vi "AdaptToInputs.vi"(3 "Term Types":T1, 4 "XRef":refnum<vi>, 5 "State In":T5) -> (0 "Reply":string[](array[string]), 2 "State Out":T5)   [LabVIEW 2018, in "Foreign Key Sort.xnode"]
uses:
  Foreign Key Sort.xnode
  State.ctl
  <vilib>/XNodeSupport/XNodeTermTypeIDPairs.ctl
  <vilib>/XNodeSupport/XNodeTermTypeIDPair.ctl
  <vilib>/XNodeSupport/XNodeType.ctl
  <vilib>/XNodeSupport/XNodeString.ctl
  <userlib>/_LAVAcr/Scripting Tools/XNode Support/TypeDefs/Array element Tests.ctl
  <userlib>/_LAVAcr/Scripting Tools/XNode Support/Find term type by ID_type.vi
  <userlib>/_LAVAcr/Scripting Tools/XNode Support/XNode Support.lvlib
  <vilib>/XNodeSupport/NI_XNodeSupport.lvlib
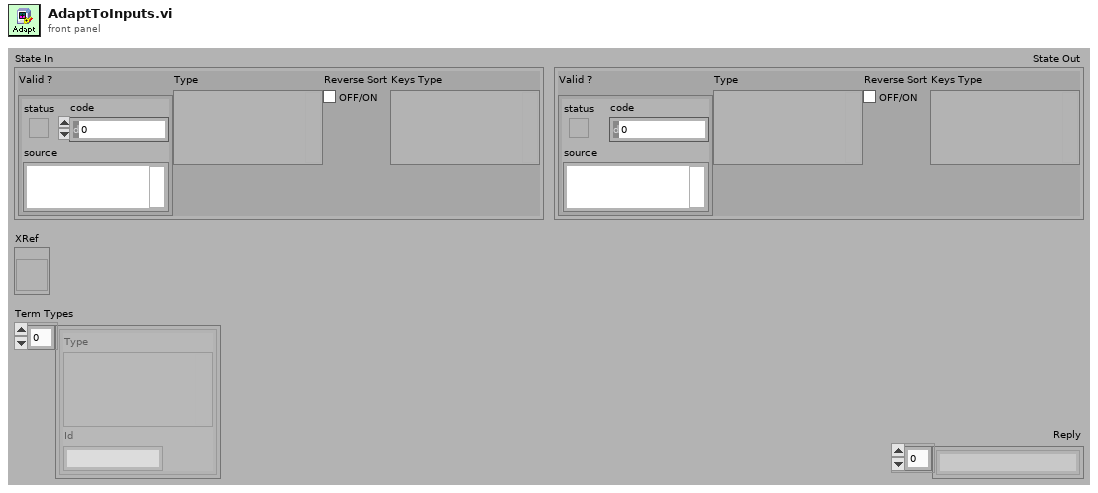
[diagram p1: front panel]
types:
  T1 = typedef "NI_XNodeSupport.lvlib/XNodeTermTypeIDPairs.ctl" = T2[]
  T2 = typedef "NI_XNodeSupport.lvlib/XNodeTermTypeIDPair.ctl" = cluster{"Type":T3, "Id":T4}
  T3 = typedef "NI_XNodeSupport.lvlib/XNodeType.ctl" = variant
  T4 = typedef "NI_XNodeSupport.lvlib/XNodeString.ctl" = string
  T5 = typedef "Foreign Key Sort.xnode/State.ctl" = cluster{"Valid ?":errorcluster, "Type":variant, "Reverse Sort":bool, "Keys Type":variant}
  T6 = enum16{"No Check", "At Least n dimensions", "Exactly N Dimensions"}
  T7 = typedef "Scripting Tools.lvlib/XNode Support.lvlib/Array element Tests.ctl" = enum16{"Any Element", "Numeric", "Integer", "Float", "Complex", "Boolean", "String", "Sortable"}
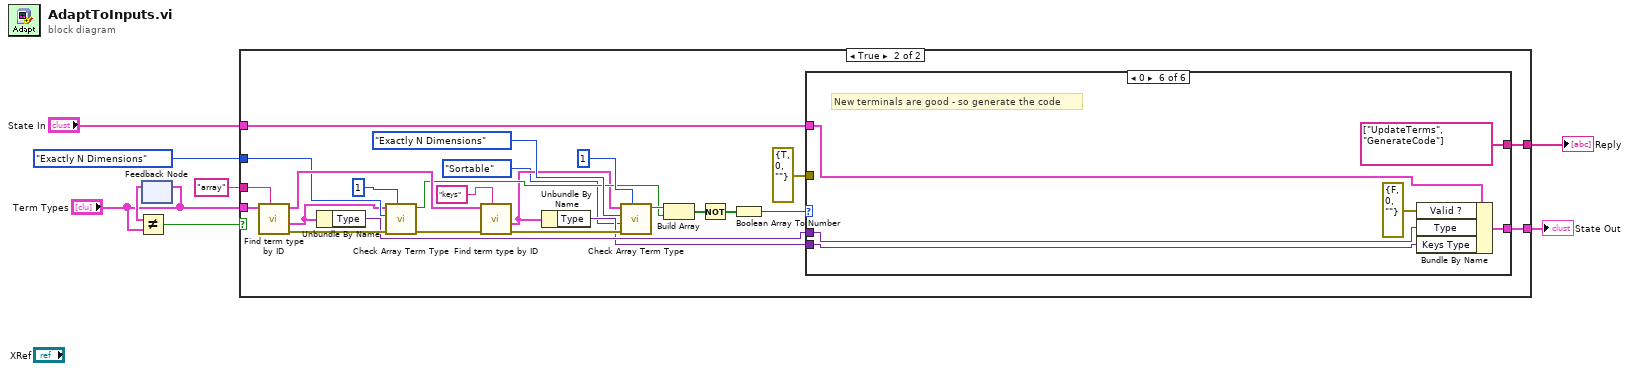
[diagram p0: block diagram]
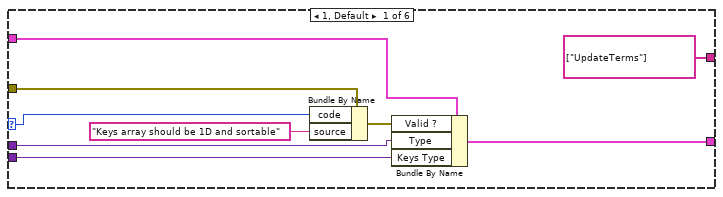
[diagram p3: hidden frame]
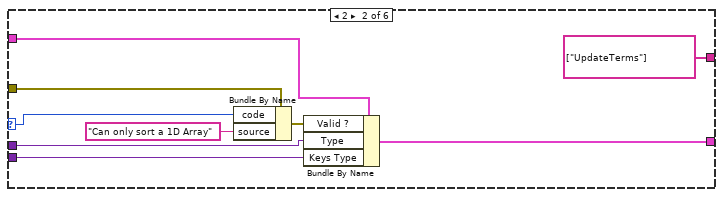
[diagram p4: hidden frame]
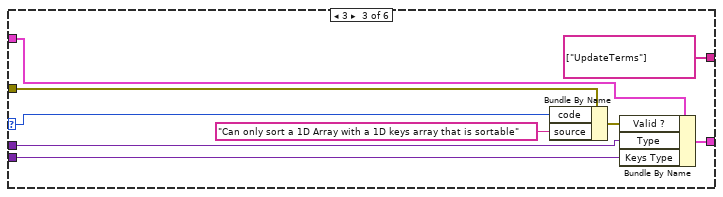
[diagram p5: hidden frame]
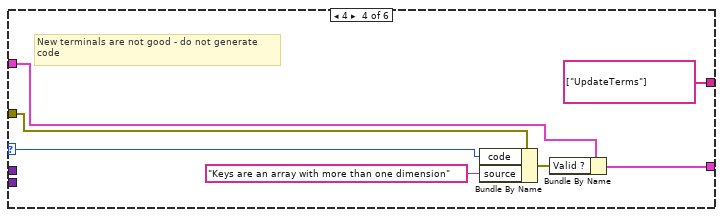
[diagram p6: hidden frame]
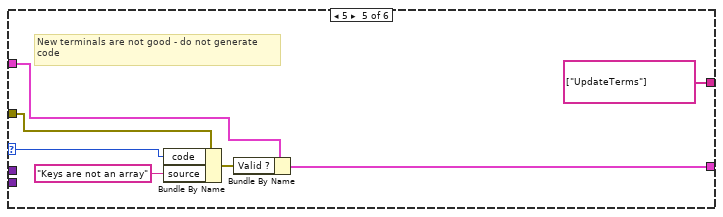
[diagram p7: hidden frame]
diagram:
  n1 = feedback-in #1("Term Types") -> ()
  n2 = feedback #1() -> (w4:T1)  [unwired: 1 out]
  n3 = Not Equal?(x=w4, y="Term Types") -> (x != y?=w1:bool)
  n4 = case shown="True" w1 {
    tunnel: [w9 w34] -> w8
    tunnel: [_ w33] -> w7
    tunnel: "array" ("Search ID") -> [_ w32]
    tunnel: T6."Exactly N Dimensions" ("Dimension Check") -> [_ w27]
    tunnel: "Term Types" -> [_ w11]
    tunnel: "State In" -> [w9 w10]
    frame False {
    }
    frame True {
      n5 = call-poly <userlib>:"Find term type by ID.vi"("Search ID"=w32, "Term Types"=w11) -> ("error out"=w28:errorcluster, "Term Type"=w16:T2, "Other Term Types"=w31:T2[])  [unwired: 1 in, 6 out]
      n6 = Unbundle By Name(w16) -> ("Type"=w15:T3)
      n7 = call <userlib>:"Check Array Term Type.vi"("Dimensions Required"=1, "error in (no error)"=w28, "Dimension Check"=w27, "Term Type"=w16) -> ("error out"=w25:errorcluster, "Is Good ?"=w20:bool)  [unwired: 1 in, 5 out]
      n8 = call-poly <userlib>:"Find term type by ID.vi"("Search ID"="keys", "error in (no error)"=w25, "Term Types"=w31) -> ("error out"=w24:errorcluster, "Term Type"=w14:T2)  [unwired: 7 out]
      n9 = Unbundle By Name(w14) -> ("Type"=w13:T3)
      n10 = call <userlib>:"Check Array Term Type.vi"("Dimensions Required"=1, "error in (no error)"=w24, "Element Check"=Array_element_Tests."Sortable", "Dimension Check"=T6."Exactly N Dimensions", "Term Type"=w14) -> ("Is Good ?"=w21:bool)  [unwired: 6 out]
      n11 = Build Array(w21, w20) -> (w19:bool[])
      n12 = Not(x=w19) -> (.not. x?=w18:bool[])
      n13 = Boolean Array To Number(Boolean array=w18) -> (number=w17:u32)
      n14 = case shown="0" w17 {
        selector: w17 -> [w37 w46 w55 w62 w69 _]
        tunnel: w10 -> [w43 w52 w61 w68 w75 w81]
        tunnel: [w42 w51 w60 w67 w74 w79] -> w34
        tunnel: [string[] ["UpdateTerms"] ("Reply") string[] ["UpdateTerms"] ("Reply") string[] ["UpdateTerms"] ("Reply") string[] ["UpdateTerms"] ("Reply") string[] ["UpdateTerms"] ("Reply") string[] ["UpdateTerms", "GenerateCode"] ("Reply")] -> w33
        tunnel: errorcluster {"status"=TRUE, "code"=0, "source"=""} ("Valid ?") -> [w40 w49 w58 w65 w72 _]
        tunnel: w13 -> [w35 w44 w53 _ _ w77]
        tunnel: w15 -> [w36 w45 w54 _ _ w76]
        frame 1, Default {
          n15 = Bundle By Name(cluster=w40, "code"=w37, "source"="Keys array should be 1D and sortable") -> (w39:errorcluster)
          n16 = Bundle By Name(cluster=w43, "Valid ?"=w39, "Type"=w36, "Keys Type"=w35) -> (w42:T5)
        }
        frame 2 {
          n17 = Bundle By Name(cluster=w49, "code"=w46, "source"="Can only sort a 1D Array") -> (w48:errorcluster)
          n18 = Bundle By Name(cluster=w52, "Valid ?"=w48, "Type"=w45, "Keys Type"=w44) -> (w51:T5)
        }
        frame 3 {
          n19 = Bundle By Name(cluster=w58, "code"=w55, "source"="Can only sort a 1D Array with a 1D keys array that is sortable") -> (w57:errorcluster)
          n20 = Bundle By Name(cluster=w61, "Valid ?"=w57, "Type"=w54, "Keys Type"=w53) -> (w60:T5)
        }
        frame 4 {
          # "New terminals are not good - do not generate\ncode"
          n21 = Bundle By Name(cluster=w65, "code"=w62, "source"="Keys are an array with more than one dimension") -> (w64:errorcluster)
          n22 = Bundle By Name(cluster=w68, "Valid ?"=w64) -> (w67:T5)
        }
        frame 5 {
          # "New terminals are not good - do not generate\ncode"
          n23 = Bundle By Name(cluster=w72, "code"=w69, "source"="Keys are not an array") -> (w71:errorcluster)
          n24 = Bundle By Name(cluster=w75, "Valid ?"=w71) -> (w74:T5)
        }
        frame 0 {
          # "New terminals are good - so generate the code"
          n25 = Bundle By Name(cluster=w81, "Valid ?"=errorcluster {"status"=FALSE, "code"=0, "source"=""}, "Type"=w76, "Keys Type"=w77) -> (w79:T5)
        }
      }
    }
  }
  "Reply" <- w7
  "State Out" <- w8
